vi "PIDloop.vi"() -> ()   [LabVIEW 2020]
uses:
  <vilib>/DAQmx/read.llb/DAQmx Read (Counter DBL 1Chan 1Samp).vi
  <vilib>/DAQmx/write.llb/DAQmx Write (Counter Frequency 1Chan 1Samp).vi
  <vilib>/DAQmx/create/channels.llb/DAQmx Create Channel (CI-Position-Angular Encoder).vi
  <vilib>/DAQmx/create/channels.llb/DAQmx Create Channel (CO-Pulse Generation-Frequency).vi
  <vilib>/DAQmx/configure/timing.llb/DAQmx Timing (Implicit).vi
  <vilib>/DAQmx/miscellaneous.llb/DAQmx Fill In Error Info.vi
  <resource>/objmgr/daqmx.rc
panel:
  out "Waveform Graph 2":dbl[][](graph)=[[0.23999999999998367, 0.23999999999998367, 0.23999999999998367, 0.19721584642224327, 0.11865958145306521, 0.05158964231075583, -0.010540642376996558, -0.042892252243967185, -0.052713476615358426, -0.05123125694428437, -0.03294735490443849, -0.019661411569368657, -0.009630300948738258, -0.0021369718376583117, 0.0027390744851638693, -0.004209444087046764, 0.003337495170998473, -0.0015583757263773472, -0.002592490281056931, 0.005295378961101709, 0.006426294110229646, -0.008237333292914976, 0.008827492399822095, -0.00998398595176442, 0.0026334995497135634, -0.004862261344458344, 0.007142748494341636, 0.0019816957625538377, -0.01106464416463584, -0.012942076987605425, -0.0021154953899040646, -0.0014014646180776393, 0.006218964476519954, 0.00015195741131147645, 0.008389461193033614, -0.0037301053784748375, 0.005302889598602272, 0.0041465516329163895, -0.006889293069070704, 0.010532629520239582, -0.014402913412553465, -0.004462335767479259, 0.0008663115564725879, 0.001410514959622246, 0.0005968271491918088, 0.004649357108337256, -0.0013277918825470812, -9.321406013826438e-05, -0.00679030498117457, 0.00013594039124770446, 0.0009793583517432186, 0.010412053974014108, -0.00931415010274601, -0.0017916633434480408, 0.0029704570658857644, 0.01099090351252942, -0.0033887942176315726, 0.008370858188597025, 0.002255697009997267, -0.000692154076162213, 0.00021625510352156545, -0.008448718016695318, -0.0014259077968092363, 0.0010683631344543757, 0.0055168324782244125, 0.006810220779596285, -0.004954215984078391, 0.010327700650813265, -0.004026871789376763, 0.0020966649537198494, -0.01392207616211057, -0.006190253764862698, 0.002417110215832453, 0.0012012138136549312, 0.0023773487413608946, -0.003077282178041687, -0.002659796130359974, 0.005624999982159551, 0.0034588572016716547, 0.0002590651077326226, -0.00876437748794097, -0.01327228104077644, -0.008705207167857833, -0.006501508250716428, 0.001698165787606843, 0.0035072266027121237, 0.011258178271989853, -0.00241507994028534, 0.01020310876667754, 0.0007788585973599236, -0.000649878437949293, -1.8940520418289983e-05, 0.0025469043178317674, 0.0032278782626733653, 0.008635178124269291, -0.010245254618946377, 0.0007560529031212931, 0.0024291909085088796, 0.004612326654523654, 0.0004589370850949178], [0.0, 0.062055359995247285, 0.1300093200052743, 0.2289433275003603, 0.2735866840707083, 0.28219470549158104, 0.2971831000650982, 0.2926658575045379, 0.28069737266394473, 0.26226849278312253, 0.25371968685757285, 0.243053837202983, 0.2679986047790973, 0.23603357694536517, 0.23319992697515346, 0.23453275887353506, 0.23665023375360156, 0.22679888143410595, 0.261026078729209, 0.22867155818058785, 0.23557236009430194, 0.2404818482883551, 0.23286340015100368, 0.23695359685739045, 0.23438634055489826, 0.2659803075473123, 0.2700926815157947, 0.2374021046265526, 0.23942052620922075, 0.22377782755164785, 0.24032338419437035, 0.22769666523237145, 0.2547702111690214, 0.2190535762009017, 0.22629930559604272, 0.25999132325542745, 0.233726902232306, 0.22797027727454683, 0.28093585572795393, 0.23380713074386233, 0.23568468663740288, 0.23986747284346563, 0.22591793388086953, 0.2579239760442477, 0.2308067956036775, 0.26359166733631306, 0.23139420281642895, 0.22813202314911707, 0.23043111530923546, 0.2277564258960087, 0.27322851903662215, 0.2331859331296318, 0.22286659249819593, 0.23158066481306117, 0.23059439243963353, 0.22692380997149011, 0.23572281017531896, 0.22789532826103062, 0.2749711832314345, 0.23932234845658643, 0.23436980601716467, 0.23842453188253473, 0.23341975225410075, 0.23971432189079556, 0.22851847632098016, 0.2294785487754327, 0.23825456440249446, 0.23325030657090845, 0.26693248231639993, 0.2636369285755564, 0.2385651626479516, 0.23444093947669745, 0.2361328884828802, 0.23031389208201553, 0.25822301233766304, 0.2382954639440497, 0.23299615095941256, 0.2198435255974891, 0.26648335346771296, 0.25925551355750265, 0.24826000505850992, 0.23133331192206547, 0.25651940769369425, 0.21073485355581148, 0.23382601925407953, 0.2187284224839877, 0.25094311460888885, 0.2224019041345908, 0.2715115923623406, 0.22050418734813482, 0.23331933648177355, 0.23364145175694007, 0.22286249465427255, 0.27859773503747404, 0.22506100727176778, 0.23295633145759537, 0.23427789941840704, 0.23302400503902243, 0.23316728201490175, 0.23392294841351094], [0.002739295745313874, 0.0, 0.0, -0.0022863185603297234, -0.004475140878330656, -0.004183462437078214, -0.0038631702030058664, -0.002022825203257132, -0.0006147671168927542, 9.423794741427015e-05, 0.0011389057650225856, 0.0008332963286027152, 0.0005580875694282342, 0.00046815985033125056, 0.0003075826556081407, -0.0004372029263119486, 0.00046832580756512335, -0.0003182344088089509, -5.82991256483676e-05, 0.0005060842265601663, 7.08657390821517e-05, -0.0009067562853390392, 0.0010795056739251873, -0.001181364318411156, 0.0007919268558501681, -0.0004158434354108137, 0.0006521909817116651, -0.0003216298528686744, -0.000808011024723058, -0.00012282748338743733, 0.0006496364725915609, 4.510777209062293e-05, 0.00042953871124013415, -0.0004006635054791652, 0.0005266784511550792, -0.000681113298772848, 0.0005622457336358155, -7.424911939692248e-05, -0.0005777880762134226, 0.0010872718722478622, -0.0015627220371675489, 0.0006019747527463882, 0.0003408248984263362, 3.051945578720987e-05, -5.107818905987364e-05, 0.0002229075153310427, -0.00037655791619468275, 7.876798070474117e-05, -0.00042297558819945596, 0.0004390769297325954, 4.457585452632882e-05, 0.0005848123445483727, -0.0012952814628217357, 0.00047022125345222904, 0.00029831865847947705, 0.0005123445450968439, -0.000895676850098081, 0.0007546675518214087, -0.00032841332363752493, -0.0001823677758261336, 5.7340376440391225e-05, -0.0005377802250409942, 0.0004408875885248504, 0.00015222483688199826, 0.0002851436685052631, 8.308675824881257e-05, -0.0007336193181073646, 0.0009678960170971374, -0.000803878693850586, 0.00034562510402402514, -0.0010015418902149455, 0.0004841199982307414, 0.000531245308123504, -7.715783689576224e-05, 6.666101365758062e-05, -0.00033593586297332105, 2.6202930285864704e-05, 0.0005493896626757942, -0.00011927993918486983, -0.00018183612398504445, -0.0005356506678863277, -0.0002842768790634494, 0.00025571522244890945, 0.00014864788282699024, 0.0004946046165546897, 0.00011689339054881106, 0.0004383784404157678, -0.0008843365636346676, 0.0006665794339898319, -0.0006204279002045846, -8.89730923802668e-05, 3.9207003365686886e-05, 0.00016715165977576106, 3.559285778543009e-05, 0.0003511744475247514, -0.0011965150235245037, 0.0006850811738555561, 0.00010484371900077604, 0.00013710408373568368, -0.00026138781009149136]]
  out "Waveform Graph":dbl[](graph)=[0.0, 0.0, 0.0, 267.40095986089574, 758.377615918292, 1177.5647355577541, 1565.879014856233, 1768.0765765248132, 1829.4592288460126, 1820.195355901799, 1705.9209681527545, 1622.8838223085625, 1560.1893809296182, 1513.3560739853654, 1482.8807844677247, 1526.309025544044, 1479.1406551812581, 1509.739848289859, 1516.203064256607, 1466.903881493112, 1459.835661811062, 1551.483333080722, 1444.8281725011082, 1562.3999121985319, 1483.540627814289, 1530.3891334028667, 1455.3578219103617, 1487.6144014840377, 1569.1540260289787, 1580.8879811725394, 1513.2218461869013, 1508.7591538629858, 1461.1314720217476, 1499.0502661793032, 1447.5658675435363, 1523.3131586154693, 1466.8569400087335, 1474.0840522942708, 1543.0580816816948, 1434.1710654984981, 1590.0182088284653, 1527.8895985467473, 1494.585552772046, 1491.1842815023604, 1496.269830317551, 1470.9415180728902, 1508.2986992659198, 1500.5825878758642, 1542.439406132344, 1499.1503725547018, 1493.8790103016045, 1434.9246626624074, 1558.2134381421665, 1511.197895896551, 1481.4346433382127, 1431.3068530466865, 1521.1799638601988, 1447.682136321265, 1485.9018936875161, 1504.3259629760141, 1498.6484056029901, 1552.8044876043493, 1508.9119237300583, 1493.3227304096597, 1465.519797011095, 1457.4361201275203, 1530.963849900492, 1435.4518709324127, 1525.1679486836065, 1486.89584403925, 1587.012976013197, 1538.6890860303945, 1484.8930611510461, 1492.4924136646562, 1485.1415703664934, 1519.2330136127619, 1516.623725814751, 1464.8437501115004, 1478.3821424895507, 1498.380843076671, 1554.7773592996348, 1582.9517565048584, 1554.4075447991152, 1540.6344265669804, 1489.3864638274565, 1478.0798337330477, 1429.6363858000586, 1515.0942496267844, 1436.230570208261, 1495.1321337665001, 1504.0617402371834, 1500.1183782526143, 1484.0818480135504, 1479.82576085829, 1446.0301367233133, 1564.0328413684192, 1495.2746693554916, 1484.8175568218185, 1471.1729584092252, 1497.1316432181566]
  out "DC":dbl=0.23412049768851437
  in  "Desired RPM":dbl=1500.0
  in  "Output Pulse Terminal":tag="/Dev1/PFI0"
  in  "B input terminal":tag="/Dev1/PFI9"
  in  "A input terminal":tag="/Dev1/PFI8"
  in  "Kd":dbl=1.0000000000000322e-07 format="%#_6p"
  in  "Ki":dbl=0.004350000000000001 format="%#_6p"
  in  "Kp":dbl=0.00015999999999998912 format="%#_6p"
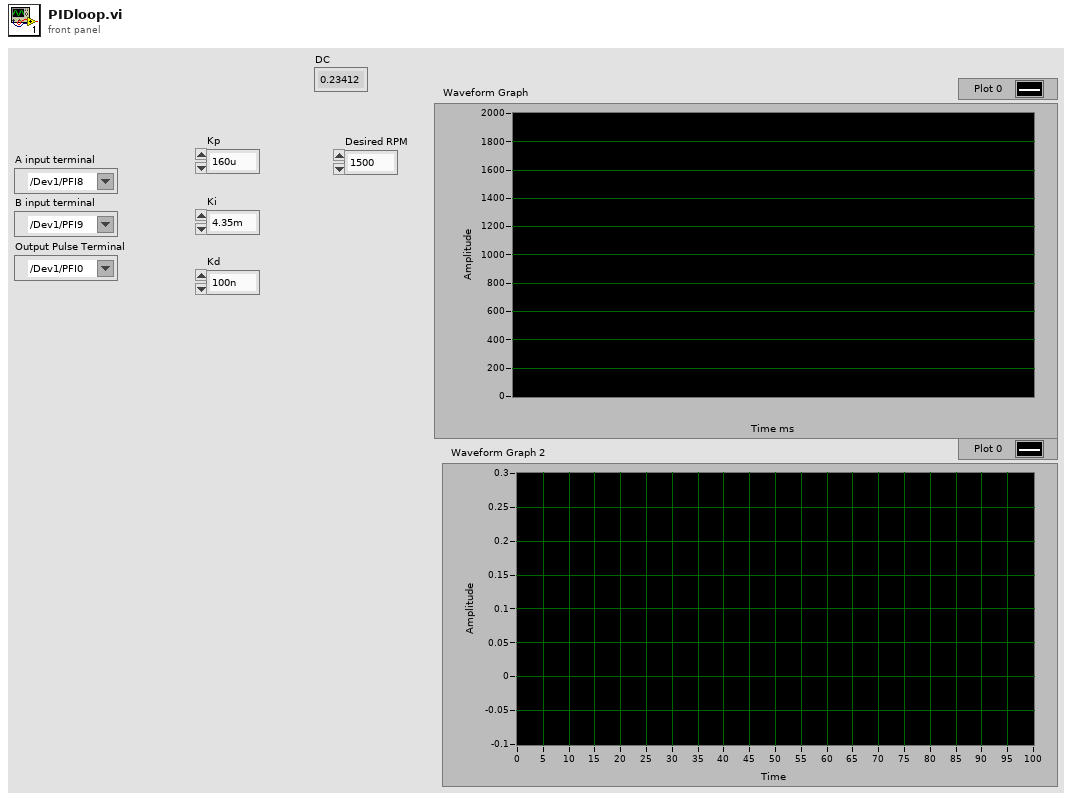
[diagram p1: front panel]
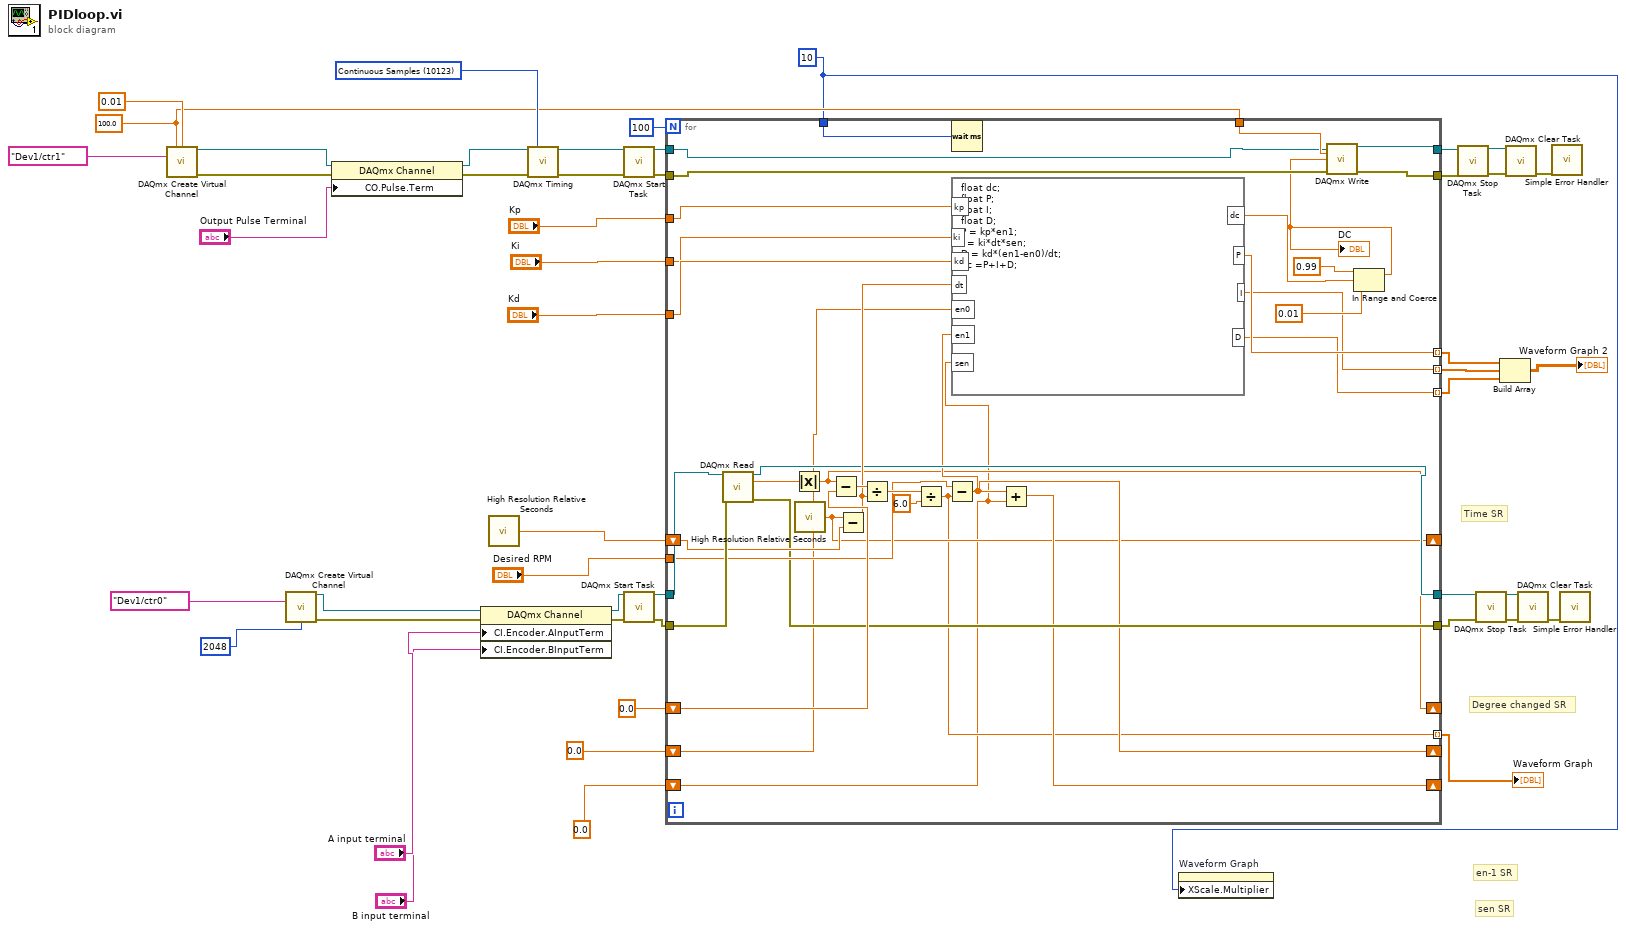
[diagram p0: block diagram]
diagram:
  w5 = u32 10 ("milliseconds to wait")
  w32 = 10123 items=["Finite Samples"=10178, "Continuous Samples"=10123, "Hardware Timed Single Point"=12522] ("sample mode")
  w19 = 100.0 ("frequency")
  # "en-1 SR"
  # "sen SR"
  # "Time SR"
  # "Degree changed SR"
  n1 = call-poly <vilib>:"DAQmx Create Virtual Channel.vi"("frequency"=w19, "duty cycle"=0.01, "counter"=tag "Dev1/ctr1") -> ("task out"=w48:refnum<k21>, "error out"=w47:errorcluster)  [unwired: 11 in]
  n2 = call-poly <vilib>:"DAQmx Create Virtual Channel.vi"("counter"=tag "Dev1/ctr0", "pulses per revolution"=u32 2048) -> ("task out"=w46:refnum<k21>, "error out"=w45:errorcluster)  [unwired: 12 in]
  n3 = property class="DAQmx Channel"(reference=w48, error in=w47, "CO.Pulse.Term"="Output Pulse Terminal") -> (reference out=w36:refnum<k21>, error out=w35:errorcluster)
  n4 = property class="DAQmx Channel"(reference=w46, error in=w45, "CI.Encoder.AInputTerm"="A input terminal", "CI.Encoder.BInputTerm"="B input terminal") -> (reference out=w44:refnum<k21>, error out=w43:errorcluster)
  n5 = call <vilib>:"High Resolution Relative Seconds.vi"() -> ("relative seconds"=w22:dbl)
  n6 = call-poly <vilib>:"DAQmx Timing.vi"("task/channels in"=w36, "sample mode"=w32, "error in"=w35) -> ("task out"=w34:refnum<k21>, "error out"=w33:errorcluster)  [unwired: 11 in]
  n7 = call <vilib>:"DAQmx Start Task.vi"("task/channels in"=w34, "error in"=w33) -> ("task out"=w30:refnum<k21>, "error out"=w29:errorcluster)  [unwired: 12 in]
  n8 = call <vilib>:"DAQmx Start Task.vi"("task/channels in"=w44, "error in"=w43) -> ("task out"=w28:refnum<k21>, "error out"=w27:errorcluster)  [unwired: 12 in]
  n9 = for {
    N: 100 -> [_]
    tunnel: "Kp" -> [w61]
    tunnel: "Ki" -> [w62]
    tunnel: "Kd" -> [w63]
    shift-right: [w56] -> _
    shift-left: w22 -> [w81]
    tunnel: "Desired RPM" -> [w74]
    shift-right: [w55] -> _
    shift-left: 0.0 -> [w79]
    tunnel: w19 -> [w73]
    shift-right: [w65] -> _
    shift-left: 0.0 -> [w66]
    shift-right: [w64] -> _
    shift-left: 0.0 -> [w49]
    tunnel: w28 -> [w83]
    tunnel: [w68] -> w9
    tunnel: w27 -> [w82]
    tunnel: [w67] -> w10
    tunnel: w30 -> [w72]
    tunnel: [w70] -> w18
    tunnel: w29 -> [w71]
    tunnel: [w69] -> w17
    tunnel: [w54] -> w6 mode=indexing
    tunnel: [w53] -> w4 mode=indexing
    tunnel: [w52] -> w3 mode=indexing
    tunnel: [w51] -> w2 mode=indexing
    tunnel: w5 -> [w50]
    n10 = call-poly <vilib>:"DAQmx Read.vi"("task/channels in"=w83, "error in"=w82) -> ("task out"=w68:refnum<k21>, "data"=w80:dbl, "error out"=w67:errorcluster)  [unwired: 11 in]
    n11 = Absolute Value(x=w80) -> (abs(x)=w55:dbl)
    n12 = call <vilib>:"High Resolution Relative Seconds.vi"() -> ("relative seconds"=w56:dbl)
    n13 = Subtract(x=w55, y=w79) -> (x-y=w78:dbl)
    n14 = Subtract(x=w56, y=w81) -> (x-y=w77:dbl)
    n15 = Divide(x=w78, y=w77) -> (x/y=w76:dbl)
    n16 = Divide(x=w76, y=6.0) -> (x/y=w54:dbl)
    n17 = Subtract(x=w74, y=w54) -> (x-y=w65:dbl)
    n18 = Wait (ms)(milliseconds to wait=w50) -> ()  [unwired: 1 out]
    n19 = formula code="float dc;\nfloat P;\nfloat I;\nfloat D;\nP = kp*en1;\nI = ki*dt*sen;\nD = kd*(en1-en0)/dt;\ndc =P+I+D;"("kp"=w61, "ki"=w62, "dt"=w77, "en0"=w66, "en1"=w65, "kd"=w63, "sen"=w49) -> ("dc"=w58:dbl, "P"=w53:dbl, "I"=w52:dbl, "D"=w51:dbl)
    n20 = Add(x=w65, y=w49) -> (x+y=w64:dbl)
    n21 = In Range and Coerce(upper limit=0.99, x=w58, lower limit=0.01) -> (coerced(x)=w57:dbl)  [unwired: 1 out]
    "DC" <- w57
    n22 = call-poly <vilib>:"DAQmx Write.vi"("task/channels in"=w72, "frequency"=w73, "duty cycle"=w57, "error in"=w71) -> ("task out"=w70:refnum<k21>, "error out"=w69:errorcluster)  [unwired: 9 in, 1 out]
  }
  "Waveform Graph" <- w6
  n23 = property on="Waveform Graph" class="WFGraph (strict)"("XScale.Multiplier"=w5) -> ()  [unwired: 2 in, 2 out]
  n24 = call <vilib>:"DAQmx Stop Task.vi"("task/channels in"=w18, "error in"=w17) -> ("task out"=w16:refnum<k21>, "error out"=w15:errorcluster)  [unwired: 12 in]
  n25 = call <vilib>:"DAQmx Stop Task.vi"("task/channels in"=w9, "error in"=w10) -> ("task out"=w13:refnum<k21>, "error out"=w12:errorcluster)  [unwired: 12 in]
  n26 = Build Array(w4, w3, w2) -> (→"Waveform Graph 2":dbl[][])
  n27 = call <vilib>:"DAQmx Clear Task.vi"("task in"=w16, "error in"=w15) -> ("error out"=w14:errorcluster)  [unwired: 13 in]
  n28 = call <vilib>:"DAQmx Clear Task.vi"("task in"=w13, "error in"=w12) -> ("error out"=w11:errorcluster)  [unwired: 13 in]
  n29 = call <vilib>:"Simple Error Handler.vi"("error in (no error)"=w14) -> ()  [unwired: 4 in, 5 out]
  n30 = call <vilib>:"Simple Error Handler.vi"("error in (no error)"=w11) -> ()  [unwired: 4 in, 5 out]
